vi "Keep position above object.vi"(7 "nr of particles":i32, 8 "bottom":dbl, 9 "right":dbl, 10 "top":dbl, 11 "left":dbl) -> (0 "Hover":bool, 1 "Roll":dbl format="%#_6f", 2 "Pitch":dbl format="%#_6f", 3 "Current Position":T1)   [LabVIEW 2014]
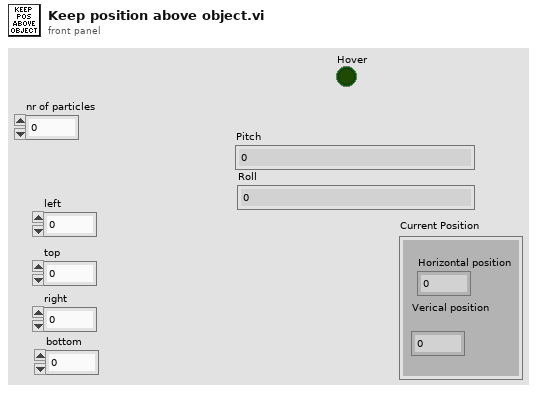
[diagram p1: front panel]
types:
  T1 = cluster{"Horizontal position":dbl, "Verical position\n":dbl}
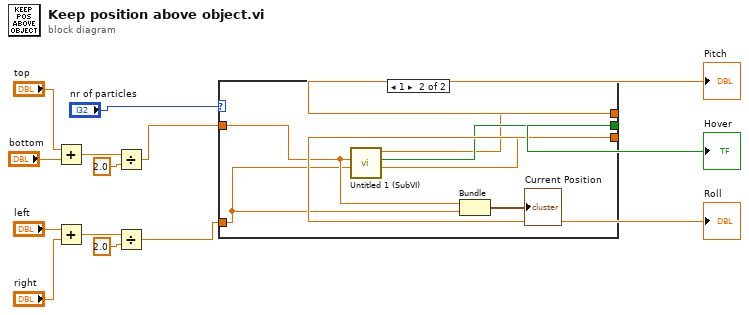
[diagram p0: block diagram]
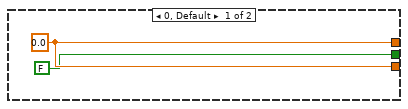
[diagram p2: hidden frame]
diagram:
  n1 = Add(x="top", y="bottom") -> (x+y=w8:dbl)
  n2 = Add(x="left", y="right") -> (x+y=w7:dbl)
  n3 = Divide(x=w8, y=2.0) -> (x/y=w6:dbl)
  n4 = Divide(x=w7, y=2.0) -> (x/y=w5:dbl)
  n5 = case shown="1" "nr of particles" {
    tunnel: w6 -> [_ w18]
    tunnel: w5 -> [_ w17]
    tunnel: [w16 w20] -> w4
    tunnel: [FALSE ("Hover") w22] -> w3
    tunnel: [w16 w19] -> w2
    frame 0, Default {
      w16 = 0.0 ("Pitch")
    }
    frame 1 {
      n6 = call "Untitled 1 (SubVI).vi"("X"=w17, "Y"=w18) -> ("Roll"=w19:dbl, "Hover"=w22:bool, "Pitch"=w20:dbl)  [unwired: 7 in]
      n7 = Bundle(w18, w17) -> (→"Current Position":cluster{dbl, dbl})  [unwired: 1 in]
    }
  }
  "Pitch" <- w4
  "Roll" <- w2
  "Hover" <- w3
